vi "Test Refresh.vi"(8 "error in (no error)":errorcluster) -> (0 "error out":errorcluster)   [LabVIEW 2019]
uses:
  <vilib>/addons/_JKI Toolkits/Caraya/classes/Test/Test.lvclass
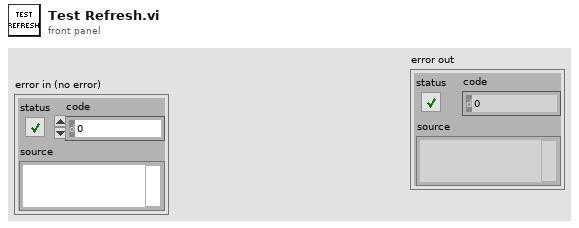
[diagram p1: front panel]
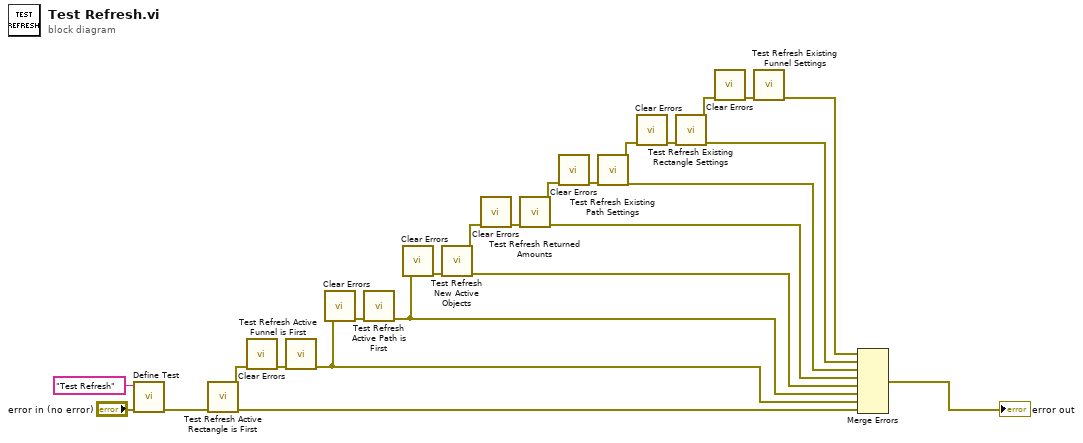
[diagram p0: block diagram]
diagram:
  n1 = call <vilib>:"Define Test.vi"("error in (no error)"="error in (no error)", "Label (VI Title)"="Test Refresh") -> ("error out"=w1:errorcluster)  [unwired: 8 in, 1 out]
  n2 = call "Test Refresh Active Rectangle is First.vi"("error in (no error)"=w1) -> ("error out"=w8:errorcluster)  [unwired: 10 in]
  n3 = call <vilib>:"Clear Errors.vi"("error in (no error)"=w8) -> ("error out"=w15:errorcluster)  [unwired: 5 in, 1 out]
  n4 = call "Test Refresh Active Funnel is First.vi"("error in (no error)"=w15) -> ("error out"=w7:errorcluster)  [unwired: 10 in]
  n5 = call <vilib>:"Clear Errors.vi"("error in (no error)"=w7) -> ("error out"=w14:errorcluster)  [unwired: 5 in, 1 out]
  n6 = call "Test Refresh Active Path is First.vi"("error in (no error)"=w14) -> ("error out"=w6:errorcluster)  [unwired: 10 in]
  n7 = call <vilib>:"Clear Errors.vi"("error in (no error)"=w6) -> ("error out"=w13:errorcluster)  [unwired: 5 in, 1 out]
  n8 = call "Test Refresh New Active Objects.vi"("error in (no error)"=w13) -> ("error out"=w5:errorcluster)  [unwired: 10 in]
  n9 = call <vilib>:"Clear Errors.vi"("error in (no error)"=w5) -> ("error out"=w12:errorcluster)  [unwired: 5 in, 1 out]
  n10 = call "Test Refresh Returned Amounts.vi"("error in (no error)"=w12) -> ("error out"=w4:errorcluster)  [unwired: 10 in]
  n11 = call <vilib>:"Clear Errors.vi"("error in (no error)"=w4) -> ("error out"=w11:errorcluster)  [unwired: 5 in, 1 out]
  n12 = call "Test Refresh Existing Path Settings.vi"("error in (no error)"=w11) -> ("error out"=w3:errorcluster)  [unwired: 10 in]
  n13 = call <vilib>:"Clear Errors.vi"("error in (no error)"=w3) -> ("error out"=w10:errorcluster)  [unwired: 5 in, 1 out]
  n14 = call "Test Refresh Existing Rectangle Settings.vi"("error in (no error)"=w10) -> ("error out"=w2:errorcluster)  [unwired: 10 in]
  n15 = call <vilib>:"Clear Errors.vi"("error in (no error)"=w2) -> ("error out"=w9:errorcluster)  [unwired: 5 in, 1 out]
  n16 = call "Test Refresh Existing Funnel Settings.vi"("error in (no error)"=w9) -> ("error out"=w16:errorcluster)  [unwired: 10 in]
  n17 = Merge Errors(w16, w2, w3, w4, w5, w6, w7, w8) -> (→"error out":errorcluster)
